vi "Write PIC SW Version.vi"(10 "PIC SW Version":string, 11 "Device in":refnum<class "PIC-Device.lvclass">) -> (3 "Device out":refnum<class "PIC-Device.lvclass">)   [LabVIEW 2020, in "PIC-Device.lvclass"]
uses:
  PIC-Device.lvclass
  PIC-Device.lvclass/PIC-Device.ctl
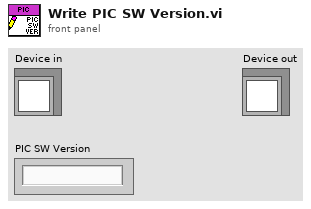
[diagram p1: front panel]
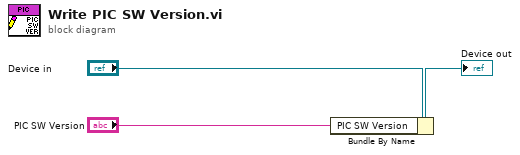
[diagram p0: block diagram]
diagram:
  n1 = Bundle By Name(cluster="Device in", "PIC SW Version"="PIC SW Version") -> (→"Device out":refnum<class "PIC-Device.lvclass">)
